vi "Receive Message.vi"(0 "ICanCommunicate In":refnum<class "Process.lvclass">, 1 "Timeout in ms (-1)":i32, 5 "ToProcessQueue":T2, 11 "Error In":errorcluster) -> (4 "ICanCommunicate Out":refnum<class "Process.lvclass">, 6 "Message":T1, 15 "Error Out":errorcluster)   [LabVIEW 2023, in "Process.lvclass"]
uses:
  Process.lvclass
  Interfaces/ICanCommunicate/ToProcessQueue.ctl
  Interfaces/ICanCommunicate/Message.ctl
  Interfaces/ICanCommunicate/ICanCommunicate.lvclass
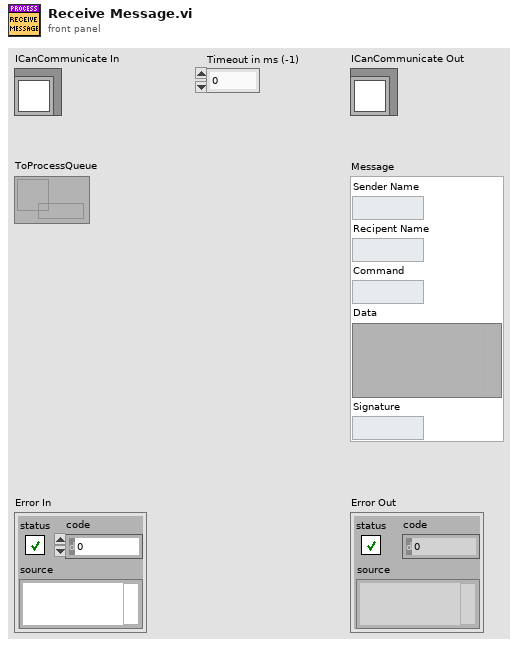
[diagram p1: front panel]
types:
  T1 = typedef "ICanCommunicate.lvclass/Message.ctl" = cluster{"Sender Name":string, "Recipent Name":string, "Command":string, "Data":variant, "Signature":string}
  T2 = typedef "ICanCommunicate.lvclass/ToProcessQueue.ctl" = refnum<queue>
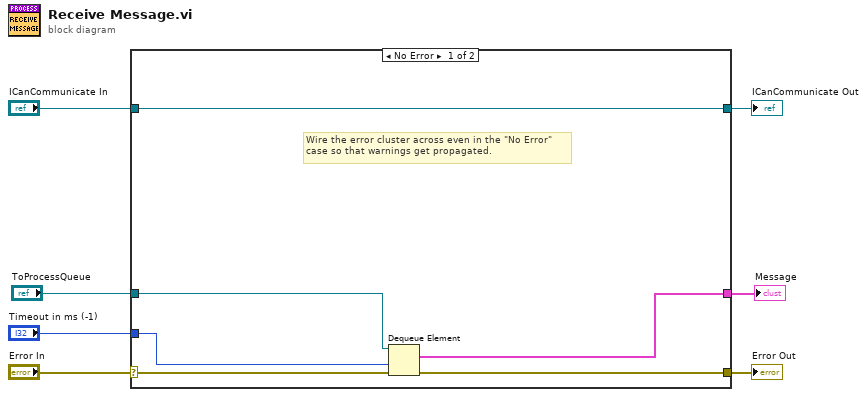
[diagram p0: block diagram]
diagram:
  n1 = case shown="No Error" "Error In" {
    selector: "Error In" -> [w12 w15]
    tunnel: [w11 w15] -> w6
    tunnel: [w13 w14] -> w4
    tunnel: "ICanCommunicate In" -> [w13 w14]
    tunnel: "Timeout in ms (-1)" -> [w10 _]
    tunnel: "ToProcessQueue" -> [w9 _]
    tunnel: [w8 _] -> w1
    frame No Error {
      # "Wire the error cluster across even in the \"No Error\"\ncase so that warnings get propagated."
      n2 = Dequeue Element(queue=w9, timeout in ms (-1)=w10, error in (no error)=w12) -> (element=w8:T1, error out=w11:errorcluster)  [unwired: 2 out]
    }
    frame Error {
    }
  }
  "Error Out" <- w6
  "ICanCommunicate Out" <- w4
  "Message" <- w1
